vi "Get_Options_without_numbers.vi"(1 "String in":string) -> (0 "after substring":string)   [LabVIEW 2020]
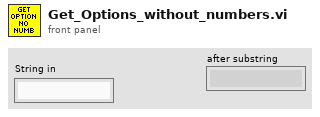
[diagram p1: front panel]
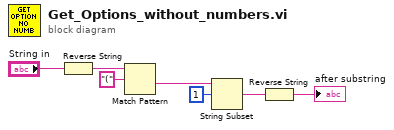
[diagram p0: block diagram]
diagram:
  n1 = Reverse String(1:"String in") -> (0:w6:string)
  n2 = Match Pattern(string=w6, regular expression="(") -> (after substring=w3:string)  [unwired: 1 in, 3 out]
  n3 = String Subset(string=w3, offset (0)=1) -> (substring=w2:string)  [unwired: 1 in]
  n4 = Reverse String(1:w2) -> (0:→"after substring":string)
